vi "dfd_Min-Max Phase Spectral Factorization (Zeros).vi"(8 "error in (no error)":errorcluster, 11 "numerator":dbl[](array[numeric])) -> (0 "error out":errorcluster, 1 "maximum phase":dbl[](array[numeric]), 2 "minimum phase":dbl[](array[numeric]))   [LabVIEW 2017, in "NI_DigFilter_Design.lvlib"]
doc: "Performs Min-Max phase spectral factorization by use of zeros of the filter."
uses:
  <vilib>/addons/Digital Filter Design/NI_DigFilter_Design.lvlib
  <vilib>/addons/Digital Filter Design/_Misc.llb/dfd_Error Cluster From Error Code (Scalar).vi
  <vilib>/Analysis/polynomials.llb/Polynomial Roots (DBL).vi
  <vilib>/addons/Digital Filter Design/NI_DigFilterLicensed.lvlib
  <vilib>/Analysis/NI_AALPro.lvlib
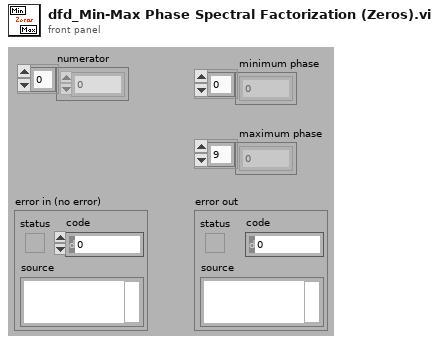
[diagram p1: front panel]
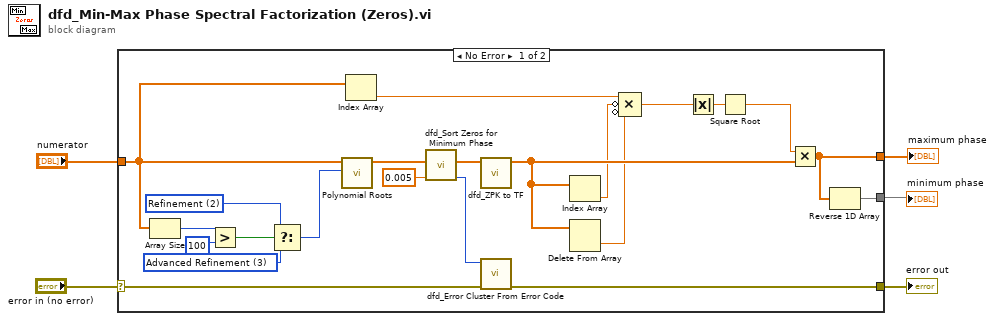
[diagram p0: block diagram]
diagram:
  n1 = case shown="No Error" "error in (no error)" {
    selector: "error in (no error)" -> [w25 w28]
    tunnel: "numerator" -> [w19 _]
    tunnel: [w7 _] -> w1
    tunnel: [w6 _] -> w2
    tunnel: [w24 w28] -> w3
    frame No Error {
      w15 = u16 2 items=["General", "Simple Classification", "Refinement", "Advanced Refinement"] ("option")
      w14 = u16 3 items=["General", "Simple Classification", "Refinement", "Advanced Refinement"] ("option")
      n2 = Array Size(array=w19) -> (size(s)=w18:i32)
      n3 = Greater?(x=w18, y=100) -> (0:w16:bool)
      n4 = Select(t=w15, s=w16, f=w14) -> (s? t:f=w13:u16)
      n5 = call-poly <vilib>:"Polynomial Roots.vi"("option"=w13, "P(x)"=w19) -> ("Roots"=w26:cdb[])  [unwired: 1 in, 8 out]
      n6 = Index Array(array=w19) -> (element=w9:dbl)  [unwired: 1 in]
      n7 = call <vilib>:"dfd_Sort Zeros for Minimum Phase.vi"("tol"=0.005, "zeros"=w26) -> ("error"=w23:i32, "zeros  in g0"=w27:cdb[])  [unwired: 1 in, 7 out]
      n8 = call <vilib>:"dfd_ZPK to TF.vi"("zeros"=w27) -> ("numerator"=w12:dbl[])  [unwired: 2 in, 8 out]
      n9 = call-poly <vilib>:"dfd_Error Cluster From Error Code.vi"("error in (no error)"=w25, "error code (0)"=w23) -> ("error out"=w24:errorcluster)  [unwired: 9 out]
      n10 = Index Array(array=w12) -> (element=w11:dbl)  [unwired: 1 in]
      n11 = Delete From Array(array=w12) -> (deleted portion=w10:dbl)  [unwired: 2 in, 1 out]
      n12 = Compound Arithmetic op=MULTIPLY(w9, invert w11, invert w10) -> (w8:dbl)
      n13 = Absolute Value(x=w8) -> (abs(x)=w22:dbl)
      n14 = Square Root(x=w22) -> (sqrt(x)=w21:dbl)
      n15 = Multiply(x=w21, y=w12) -> (x*y=w7:dbl[])
      n16 = Reverse 1D Array(array=w7) -> (reversed array=w6:dbl[])
    }
    frame Error {
    }
  }
  "minimum phase" <- w2
  "maximum phase" <- w1
  "error out" <- w3
